vi "rotate_while_checking.vi"(8 "degrees to  rotate":dbl, 9 "right(T)/left(F)":bool, 10 "power":u16=75, 11 "NXT 2":T1={"Hardware"="NXT", "Flattened String"=""}) -> (0 "fail":bool, 1 "degrees rotated":dbl, 3 "NXT":T1={"Hardware"="NXT", "Flattened String"=""})   [LabVIEW 2012]
uses:
  <vilib>/NXT/Subs/LVHSConnector.ctl
  <vilib>/NXT/Subs/MotorOutput.ctl
  <vilib>/NXT/Dual Mode Library/Motors/MotorBrake.vi
  <vilib>/NXT/Dual Mode Library/Display/drawNumber.vi
  <vilib>/NXT/Dual Mode Library/Waits/Wait_Num(msec).vi
  <vilib>/NXT/Dual Mode Library/Motors/MotorOn.vi
  <vilib>/NXT/Dual Mode Library/Motors/MotorReverse.vi
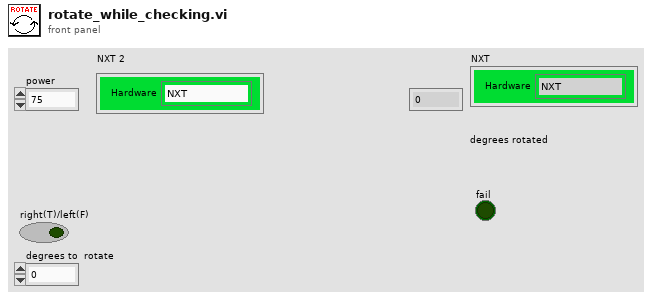
[diagram p1: front panel]
types:
  T1 = typedef "LVHSConnector.ctl" = cluster{"Hardware":string, "Flattened String":string}
  T2 = typedef "MotorOutput.ctl" = u8
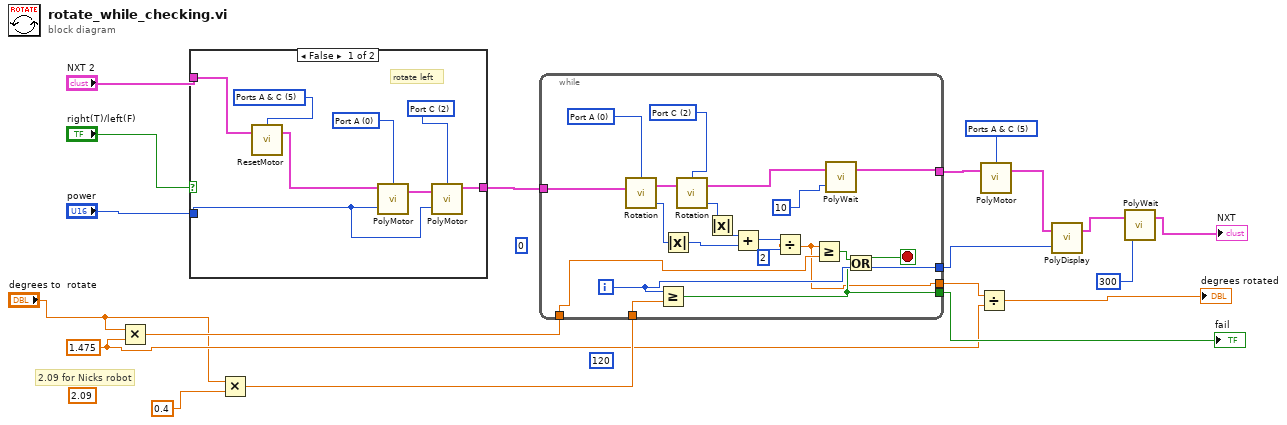
[diagram p0: block diagram]
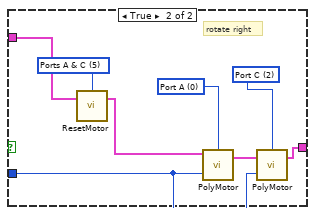
[diagram p2: hidden frame]
diagram:
  (unwired) i16 120 ("y")
  (unwired) i64 0 ("y")
  w6 = 1.475 ("Max Value")
  (unwired) 2.09 ("Max Value")
  w14 = T2 5 items=["Port A"=0, "Port B"=1, "Port C"=2, "Ports A & B"=4, "Ports A & C"=5, "Ports B & C"=6, "All Ports"=3] ("Port (All Ports)")
  # "2.09 for Nicks robot"
  n1 = Multiply(x="degrees to  rotate", y=w6) -> (x*y=w13:dbl)
  n2 = case shown="False" "right(T)/left(F)" {
    tunnel: "power" -> [w20 w28]
    tunnel: "NXT 2" -> [w24 w30]
    tunnel: [w22 w29] -> w17
    frame False {
      w21 = T2 5 items=["Port A"=0, "Port B"=1, "Port C"=2, "Ports A & B"=4, "Ports A & C"=5, "Ports B & C"=6, "All Ports"=3] ("Port (All Ports)")
      w27 = T2 2 items=["Port A"=0, "Port B"=1, "Port C"=2, "Ports A & B"=4, "Ports A & C"=5, "Ports B & C"=6, "as"=3] ("Output Port (All Ports)")
      w25 = T2 0 items=["Port A"=0, "Port B"=1, "Port C"=2, "Ports A & B"=4, "Ports A & C"=5, "Ports B & C"=6, "as"=3] ("Output Port (All Ports)")
      # "rotate left"
      n3 = call <vilib>:"ResetMotor.vi"("NXT"=w24, "Port (All Ports)"=w21) -> ("NXT"=w23:T1)  [unwired: 2 in]
      n4 = call-poly <vilib>:"PolyMotor.vi"("Power (75)"=w20, "NXT"=w23, "Output Port (All Ports)"=w25) -> ("NXT"=w26:T1)  [unwired: 1 in]
      n5 = call-poly <vilib>:"PolyMotor.vi"("Power (75)"=w20, "NXT"=w26, "Output Port (All Ports)"=w27) -> ("NXT"=w22:T1)  [unwired: 1 in]
    }
    frame True {
      w31 = T2 5 items=["Port A"=0, "Port B"=1, "Port C"=2, "Ports A & B"=4, "Ports A & C"=5, "Ports B & C"=6, "All Ports"=3] ("Port (All Ports)")
      w35 = T2 2 items=["Port A"=0, "Port B"=1, "Port C"=2, "Ports A & B"=4, "Ports A & C"=5, "Ports B & C"=6, "as"=3] ("Output Port (All Ports)")
      w33 = T2 0 items=["Port A"=0, "Port B"=1, "Port C"=2, "Ports A & B"=4, "Ports A & C"=5, "Ports B & C"=6, "as"=3] ("Output Port (All Ports)")
      # "rotate right"
      n6 = call <vilib>:"ResetMotor.vi"("NXT"=w30, "Port (All Ports)"=w31) -> ("NXT"=w32:T1)  [unwired: 2 in]
      n7 = call-poly <vilib>:"PolyMotor.vi"("Power (75)"=w28, "NXT"=w32, "Output Port (All Ports)"=w33) -> ("NXT"=w34:T1)  [unwired: 1 in]
      n8 = call-poly <vilib>:"PolyMotor.vi"("Power (75)"=w28, "NXT"=w34, "Output Port (All Ports)"=w35) -> ("NXT"=w29:T1)  [unwired: 1 in]
    }
  }
  n9 = Multiply(x="degrees to  rotate", y=0.4 ("Max Value")) -> (x*y=w10:dbl)
  n10 = while {
    tunnel: w17 -> [w55]
    tunnel: w13 -> [w45]
    tunnel: [w43] -> w15
    tunnel: w10 -> [w39]
    tunnel: [w38] -> w8
    tunnel: [w37] -> w9
    tunnel: [w36] -> w7
    i -> [w38]
    stop <- w40 stop-if-true
    w52 = T2 2 items=["Port A"=0, "Port B"=1, "Port C"=2, "Ports A & B"=4, "Ports A & C"=5, "Ports B & C"=6, "as"=3] ("Output Port (All Ports)")
    w53 = T2 0 items=["Port A"=0, "Port B"=1, "Port C"=2, "Ports A & B"=4, "Ports A & C"=5, "Ports B & C"=6, "as"=3] ("Output Port (All Ports)")
    n11 = call <vilib>:"Rotation.vi"("NXT"=w55, "Port (Port A)"=w53) -> ("Angle of Rotation"=w51:i32, "NXT"=w54:T1)  [unwired: 1 in]
    n12 = Greater Or Equal?(x=w38, y=w39) -> (x >= y?=w37:bool)
    n13 = Absolute Value(x=w51) -> (abs(x)=w49:i32)
    n14 = call <vilib>:"Rotation.vi"("NXT"=w54, "Port (Port A)"=w52) -> ("Angle of Rotation"=w50:i32, "NXT"=w44:T1)  [unwired: 1 in]
    n15 = Absolute Value(x=w50) -> (abs(x)=w48:i32)
    n16 = Add(x=w48, y=w49) -> (x+y=w47:i32)
    n17 = Divide(x=w47, y=2) -> (x/y=w36:dbl)
    n18 = Greater Or Equal?(x=w36, y=w45) -> (x >= y?=w41:bool)
    n19 = call-poly <vilib>:"PolyWait.vi"("Time (100 msec)"=10 ("y"), "NXT"=w44) -> ("NXT"=w43:T1)  [unwired: 2 in]
    n20 = Or(x=w41, y=w37) -> (x .or. y?=w40:bool)
  }
  "fail" <- w9
  n21 = Divide(x=w7, y=w6) -> (x/y=→"degrees rotated":dbl)
  n22 = call-poly <vilib>:"PolyMotor.vi"("NXT"=w15, "Port (All Ports)"=w14) -> ("NXT"=w12:T1)  [unwired: 2 in]
  n23 = call-poly <vilib>:"PolyDisplay.vi"("number"=w8, "NXT"=w12) -> ("NXT"=w3:T1)  [unwired: 2 in]
  n24 = call-poly <vilib>:"PolyWait.vi"("Time (100 msec)"=i16 300 ("y"), "NXT"=w3) -> ("NXT"=→"NXT":T1)  [unwired: 2 in]
